vi "TCPIP.vi"() -> ()   [LabVIEW 2015]
uses:
  Galobal variable_TI.vi
panel:
  in  "mode (standard)":T1(ring)=enum."CRLF"
  out "concatenated string":string
  in  "Client Closed":string="The client VI closed the connection."
  in  "Stop":bool
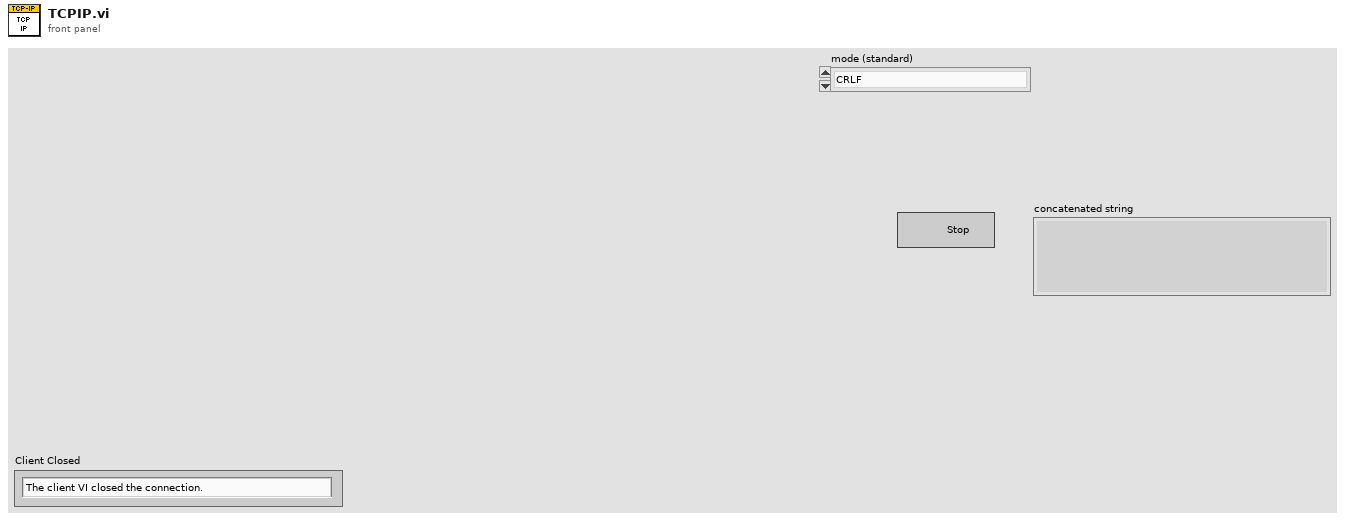
[diagram p1: front panel]
types:
  T1 = enum16{"Standard", "Buffered", "CRLF", "Immediate"}
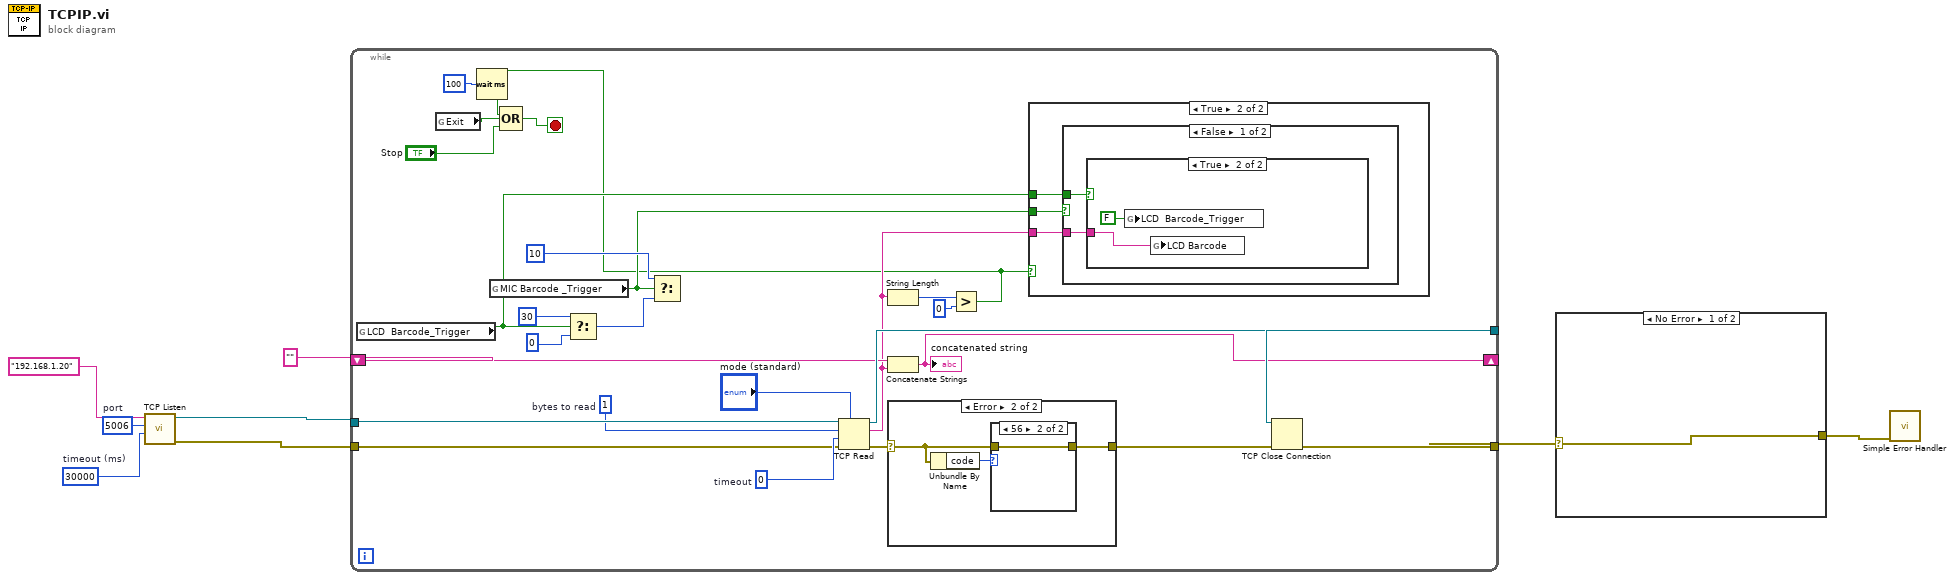
[diagram p0: block diagram]
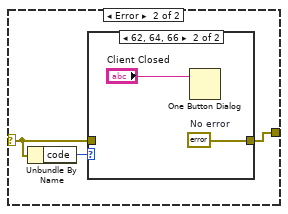
[diagram p2: hidden frame]
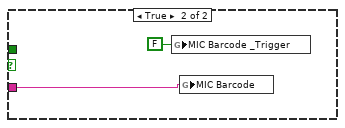
[diagram p6: hidden frame]
diagram:
  w5 = u16 5006  # port
  w6 = 30000  # timeout (ms)
  n1 = call <vilib>:"TCP Listen.vi"("timeout ms (wait forever: -1)"=w6, "port"=w5, "service name"="192.168.1.20") -> ("error out"=w2:errorcluster, "connection ID"=w3:refnum<k5>)  [unwired: 4 in, 3 out]
  n2 = while {
    tunnel: [w29] -> w9
    tunnel: [w32] -> w10
    tunnel: w3 -> [w28]
    tunnel: w2 -> [w27]
    shift-right: [w24] -> _
    shift-left: "" -> [w25]
    stop <- w33 stop-if-true
    w31 = 0  # timeout
    w11 = 1  # bytes to read
    # "TCP Server Loop"
    n3 = global read "Galobal variable_TI.vi" "LCD  Barcode_Trigger"() -> (w15:bool)
    n4 = global read "Galobal variable_TI.vi" "Exit"() -> (w21:bool)
    n5 = Wait (ms)(milliseconds to wait=u32 100) -> ()  [unwired: 1 out]
    n6 = global read "Galobal variable_TI.vi" "MIC Barcode _Trigger"() -> (w14:bool)
    n7 = Select(t=30, s=w15, f=0) -> (s? t:f=w18:i32)
    n8 = Select(t=10, s=w14, f=w18) -> ()  [unwired: 1 out]
    n9 = TCP Read(connection ID=w28, bytes to read=w11, error in (no error)=w27, 7:"mode (standard)", 9:w31) -> (connection ID out=w32:refnum<k5>, data out=w20:string, error out=w30:errorcluster)
    n10 = String Length(string=w20) -> (length=w23:i32)
    n11 = Concatenate Strings(w25, w20) -> (w24:string)
    "concatenated string" <- w24
    n12 = case shown="Error" w30 {
      selector: w30 -> [w44 w46]
      tunnel: [w44 w45] -> w29
      frame No Error {
      }
      frame Error {
        n13 = Unbundle By Name(w46) -> ("code"=w47:i32)
        n14 = case shown="56" w47 {
          tunnel: w46 -> [w48 w49]
          tunnel: [w48 w49] -> w45
          frame Default {
          }
          frame 56 {
          }
        }
      }
    }
    n15 = Greater?(x=w23, y=0) -> (0:w13:bool)
    n16 = Compound Arithmetic op=OR(w13, w21, "Stop") -> (w33:bool)
    n17 = case shown="True" w13 {
      tunnel: w20 -> [_ w37]
      tunnel: w15 -> [_ w36]
      tunnel: w14 -> [_ w35]
      frame False {
      }
      frame True {
        n18 = case shown="False" w35 {
          tunnel: w37 -> [w39 w43]
          tunnel: w36 -> [w38 _]
          frame False {
            n19 = case shown="True" w38 {
              tunnel: w39 -> [_ w40]
              frame False {
              }
              frame True {
                n20 = global write "Galobal variable_TI.vi" "LCD  Barcode_Trigger"(FALSE ("LCD  Barcode_Trigger")) -> ()
                n21 = global write "Galobal variable_TI.vi" "LCD Barcode"(w40) -> ()
              }
            }
          }
          frame True {
            n22 = global write "Galobal variable_TI.vi" "MIC Barcode _Trigger"(FALSE ("MIC Barcode _Trigger")) -> ()
            n23 = global write "Galobal variable_TI.vi" "MIC Barcode"(w43) -> ()
          }
        }
      }
    }
  }
  n24 = TCP Close Connection(connection ID=w10, error in (no error)=w9) -> (error out=w8:errorcluster)  [unwired: 2 out]
  n25 = case shown="No Error" w8 {
    selector: w8 -> [w50 w52]
    tunnel: [w50 w51] -> w7
    frame No Error {
    }
    frame Error {
      n26 = Unbundle By Name(w52) -> ("code"=w53:i32)
      n27 = case shown="62, 64, 66" w53 {
        tunnel: w52 -> [w54 _]
        tunnel: [w54 w56] -> w51
        frame Default {
        }
        frame 62, 64, 66 {
          w56 = errorcluster {"status"=FALSE, "code"=0, "source"=""}  # No error
          n28 = One Button Dialog(message="Client Closed") -> ()  [unwired: 1 in, 1 out]
        }
      }
    }
  }
  n29 = call <vilib>:"Simple Error Handler.vi"("error in (no error)"=w7) -> ()  [unwired: 1 in, 8 out]
